vi "Sensor_vorne_rechts.vi"() -> (3 "Abstand in cm":dbl(knob)=68.0 scale=5.0..160.0)   [LabVIEW 2016]
doc: "SubVI liest IR Sensor aus und berechnet Servo-Wert anhand der erstellten Kurve\n05.04.17_Tloe"
uses:
  <vilib>/myRIO/Instrument Drivers/Onboard IO/AI/typedefs/AI Reference.ctl
  <vilib>/myRIO/Common/Instrument Driver Framework/Utilities/typedefs/myRIO Generic Hardware Reference.ctl
  <vilib>/myRIO/Common/Instrument Driver Framework/Utilities/typedefs/Hardware Version Enum.ctl
  <vilib>/myRIO/Common/Instrument Driver Framework/Utilities/typedefs/myRIO v1.0 Reference.ctl
  <vilib>/myRIO/Common/Instrument Driver Framework/Utilities/typedefs/Generic FPGA Reference.ctl
  <vilib>/myRIO/Common/Instrument Driver Framework/myRIO v1.0/AI/typedefs/AI Channels List.ctl
  <vilib>/myRIO/Common/Instrument Driver Framework/myRIO v1.0/AI/typedefs/AI Channels Enum.ctl
  <vilib>/myRIO/Common/Instrument Driver Framework/Utilities/typedefs/Analog Scaling Constants List.ctl
  <vilib>/myRIO/Common/Instrument Driver Framework/Utilities/typedefs/Analog Scaling Constants.ctl
  <vilib>/userdefined/High Color/nirio_resource_hc.ctl
  <vilib>/myRIO/Instrument Drivers/Onboard IO/AI/vis/Read.vi
  <vilib>/myRIO/Common/Instrument Driver Framework/myRIO v1.0/AI/vis/myRIO v1.1 Open AI.vi
  <vilib>/myRIO/Common/Instrument Driver Framework/Utilities/vis/Is FPGA Ref Available.vi
  <vilib>/myRIO/Common/Instrument Driver Framework/Utilities/vis/Validate Channels.vi
  <vilib>/myRIO/Common/Instrument Driver Framework/myRIO v1.0/AI/vis/myRIO v1.0 Reserve AI.vi
  <vilib>/myRIO/Common/Instrument Driver Framework/myRIO v1.0/AI/vis/myRIO v1.0 Build MUX Configuration AI.vi
  <vilib>/myRIO/Common/Instrument Driver Framework/myRIO v1.0/Resource Manager/vis/myRIO v1.0 Reserve Channel List.vi
  <vilib>/myRIO/Common/Instrument Driver Framework/myRIO v1.0/Resource Manager/vis/myRIO v1.0 Reserve Channel.vi
  <vilib>/myRIO/Common/Instrument Driver Framework/myRIO v1.0/Resource Manager/vis/myRIO v1.0 Unreserve Channel.vi
  <vilib>/myRIO/Common/Instrument Driver Framework/myRIO v1.0/Resource Manager/vis/myRIO v1.0 Build Mutex Name.vi
  <vilib>/myRIO/Common/Instrument Driver Framework/myRIO v1.0/AI/vis/myRIO v1.0 Read AI.vi
  <vilib>/Utility/error.llb/Error Cluster From Error Code.vi
  <vilib>/myRIO/Common/Instrument Driver Framework/myRIO v1.0/myRIO v1.0 Close.vi
  <vilib>/myRIO/Common/Instrument Driver Framework/Utilities/vis/IO Manager.vi
  <vilib>/myRIO/Common/Instrument Driver Framework/Utilities/vis/Configuration Manager.vi
  <vilib>/myRIO/Common/Instrument Driver Framework/myRIO v1.0/AI/vis/myRIO v1.0 Get Scaling Constants AI.vi
  <vilib>/myRIO/Common/Instrument Driver Framework/myRIO v1.0/myRIO v1.1 Open.vi
  <vilib>/Utility/VariantDataType/GetNumericInfo.vi
  <vilib>/myRIO/Instrument Drivers/Onboard IO/AI/vis/myRIO AI Open.xnode
  <vilib>/myRIO/Express VI/Onboard IO/AI/AI Express VI.xnode
  <vilib>/myRIO/Instrument Drivers/Onboard IO/AI/AI.lvlib
  <vilib>/ptbypt/NI_PtbyPt.lvlib
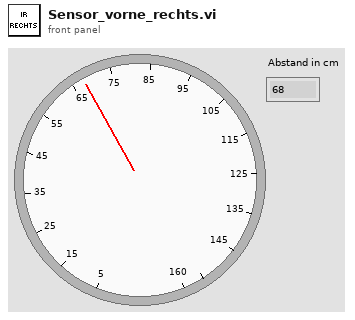
[diagram p1: front panel]
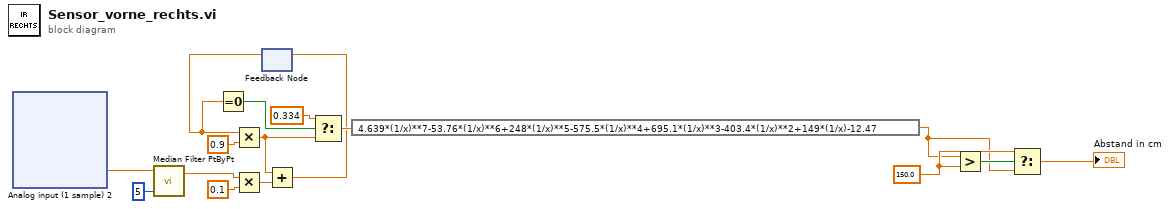
[diagram p0: block diagram]
diagram:
  w3 = 150.0 ("y")
  n1 = xnode "Analog input (1 sample) 2"() -> ("B/AI3 (Pin 9)"=w7:dbl)  [unwired: 1 in, 1 out]
  n2 = call <vilib>:"Median Filter PtByPt.vi"("rank"=5, "x"=w7) -> ("Filtered x"=w6:dbl)  [unwired: 2 in, 1 out]
  n3 = Multiply(x=w6, y=0.1) -> (x*y=w14:dbl)
  n4 = feedback #1() -> (w8:dbl)  [unwired: 1 in]
  n5 = Equal To 0?(x=w8) -> (x = 0?=w13:bool)
  n6 = Multiply(x=w8, y=0.9) -> (x*y=w10:dbl)
  n7 = Add(x=w10, y=w14) -> (x+y=w9:dbl)
  n8 = feedback-in #1(w9) -> ()
  n9 = Select(t=0.334, s=w13, f=w10) -> (s? t:f=w11:dbl)
  n10 = expression code="4.639*(1/x)**7-53.76*(1/x)**6+248*(1/x)**5-575.5*(1/x)**4+695.1*(1/x)**3-403.4*(1/x)**2+149*(1/x)-12.47"(w11) -> (w2:dbl)
  n11 = Greater?(x=w2, y=w3) -> (0:w4:bool)
  n12 = Select(t=w3, s=w4, f=w2) -> (s? t:f=→"Abstand in cm":dbl)
